vi "setVoltage.vi"(8 "error in (no error)":errorcluster, 9 "Voltage in Volts (1)":dbl=1.0 format="%#_13g", 10 "Channel Nr (1)":string="1", 11 "VISA resource name":refnum<visa-resource-name>) -> (0 "error out":errorcluster, 3 "VISA resource name out":refnum<visa-resource-name>)   [LabVIEW 2023, in "Tti-Pl303Qmd.lvlib"]
doc: "Set Voltage of Channel"
uses:
  Tti-Pl303Qmd.lvlib
  <vilib>/Utility/error.llb/Error Cluster From Error Code.vi
  <vilib>/ErrorRing/Error Ring.xnode
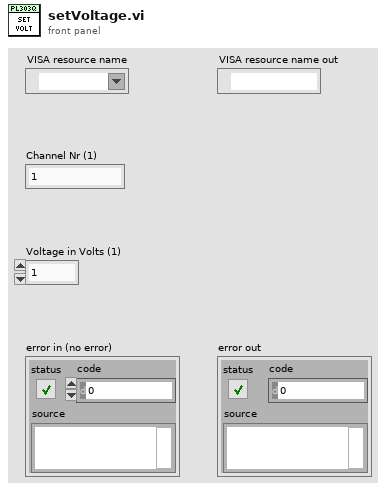
[diagram p1: front panel]
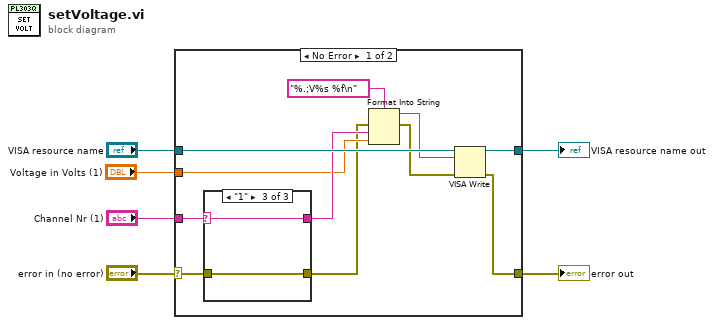
[diagram p0: block diagram]
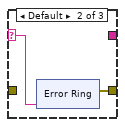
[diagram p3: hidden frame]
diagram:
  n1 = case shown="No Error" "error in (no error)" {
    selector: "error in (no error)" -> [w14 w32]
    tunnel: "VISA resource name" -> [w16 w31]
    tunnel: [w17 w32] -> w6
    tunnel: "Channel Nr (1)" -> [w15 _]
    tunnel: "Voltage in Volts (1)" -> [w11 _]
    tunnel: [w7 w31] -> w2
    frame No Error {
      n2 = case shown="\"1\"" w15 {
        selector: w15 -> [w19 w20 w29]
        tunnel: w14 -> [w18 _ w30]
        tunnel: [w18 w21 w30] -> w10
        tunnel: [w19 _ w29] -> w12
        frame "2" {
        }
        frame Default {
          n3 = xnode "Error Ring"("parameter 0"=w20) -> ("error out"=w21:errorcluster)
        }
        frame "1" {
        }
      }
      n4 = Format Into String(format string="%.;V%s %f\n" ("write buffer"), error in=w10, w12, w11) -> (resulting string=w8:string, error out=w9:errorcluster)  [unwired: 1 in]
      n5 = VISA Write(VISA resource name=w16, write buffer=w8, error in (no error)=w9) -> (VISA resource name out=w7:refnum<visa-resource-name>, error out=w17:errorcluster)  [unwired: 1 out]
    }
    frame Error {
    }
  }
  "error out" <- w6
  "VISA resource name out" <- w2
